vi "JSON Serialization error handler.vi"(8 "error in (no error)":errorcluster, 10 "Error check path index":u64, 11 "Previous path error string":string) -> (0 "error out":errorcluster, 1 "errorInString?":bool, 2 "Concaternated error\nstring":string, 3 "No error?":bool)   [LabVIEW 2015]
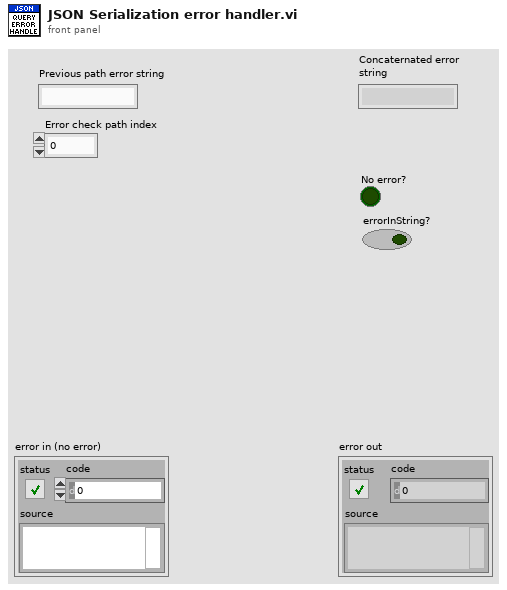
[diagram p1: front panel]
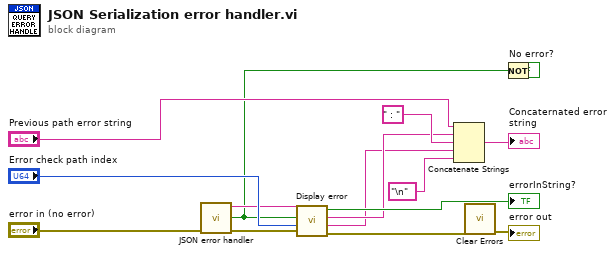
[diagram p0: block diagram]
diagram:
  n1 = call "JSON error handler.vi"("error constant"="error in (no error)") -> ("error out"=w4:errorcluster, "Error?"=w2:bool, "Error message out"=w3:string)  [unwired: 8 in]
  n2 = call "Display error.vi"("error in (no error)"=w4, "error path index in"="Error check path index", "error?"=w2, "string check in"=w3) -> ("error out"=w9:errorcluster, "string check"=w11:string, "path index"=w12:string, "errorInString?"=→"errorInString?":bool)  [unwired: 4 in]
  n3 = Concatenate Strings("Previous path error string", w12, " : " ("string"), w11, "\n" ("string")) -> (→"Concaternated error\nstring":string)
  n4 = call <vilib>:"Clear Errors.vi"("error in (no error)"=w9) -> ("error out"=→"error out":errorcluster)  [unwired: 5 in, 1 out]
  n5 = Not(x=w2) -> (.not. x?=→"No error?":bool)
